vi "GraphsUpdateMain.vi"(0 "raw graph ref":refnum<vi>, 1 "File Paths":T2={"Local Save Path"=path "\\\\smbhome.uscs.susx.ac.uk\\cv222/Desktop/data", "Newton Save Path"=path "Z:/#Projects/Entanglement/data", "File Name"="test", "LocalSave"=TRUE}, 3 "Compiler Settings":T1={"Python Path"=path "", "Main File"="mainscript.py", "Meta File"="metascript.txt", "Aux File"="auxscript.py", "Pre File"="metascript.txt"}, 5 "mean graph ref":refnum<vi>, 7 "proc graph ref":refnum<vi>, 9 "ControllerSettingsRef":refnum<vi>, 11 "error in (no error)":errorcluster) -> (15 "error out":errorcluster)   [LabVIEW 2019]
uses:
  controls/FilePaths.ctl
  PulseCompiler/CompilerSettings.ctl
  controls/ControllerSettings.ctl
  controls/GlobalExp.vi
  Global.lvlib
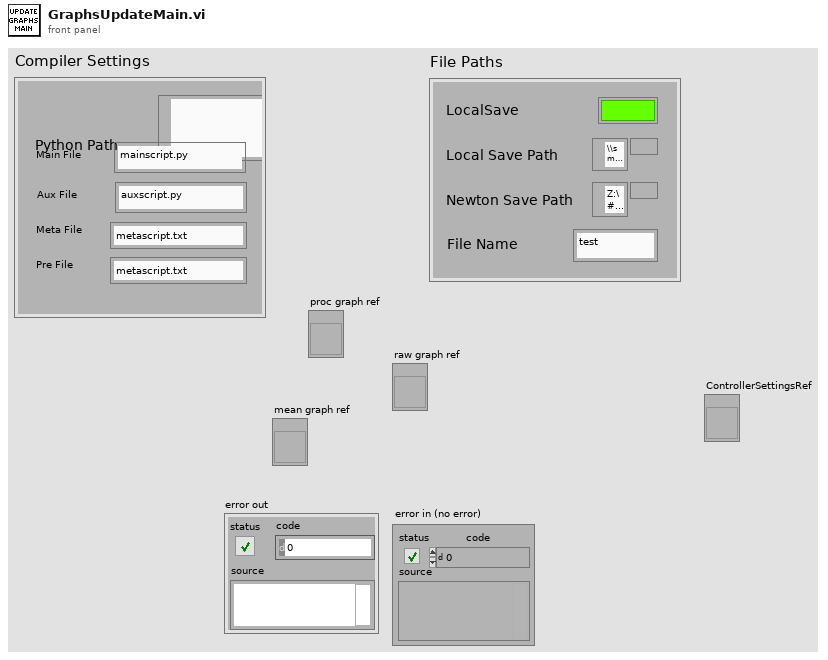
[diagram p1: front panel]
types:
  T1 = typedef "CompilerSettings.ctl" = cluster{"Python Path":path, "Main File":string, "Meta File":string, "Aux File":string, "Pre File":string}
  T2 = typedef "FilePaths.ctl" = cluster{"Local Save Path":path, "Newton Save Path":path, "File Name":string, "LocalSave":bool}
  T3 = typedef "MasterExpControl.ctl" = cluster{"Main Steps":dbl, "Main Runs":dbl, "ExpStatus":enum16{"Innit", "Stop", "Idle", "MainRunning", "AuxRunning"}, "Main Current Step":dbl, "ExpNum":dbl, "NewData":bool, "date":string, "command":string, "Stop":bool, "Pause":bool, "Mathematica":string, "Main/Meta":bool, "UpdateMath":bool, "Camera":bool, "MetaExpOver":bool, "NextMetaExp":bool}
  T4 = typedef "ControllerSettings.ctl" = cluster{"Aux Sequence":bool, "Camera":bool, "Recrystallize":bool, "Raw graph":bool, "Mean graph":bool, "Calculate probs":bool, "Find fit":bool, "ReX Time [s] :":dbl, "Lock Voltage :":dbl, "Line trig ":bool, "Check Fluo":bool, "Pre Sequence":bool}
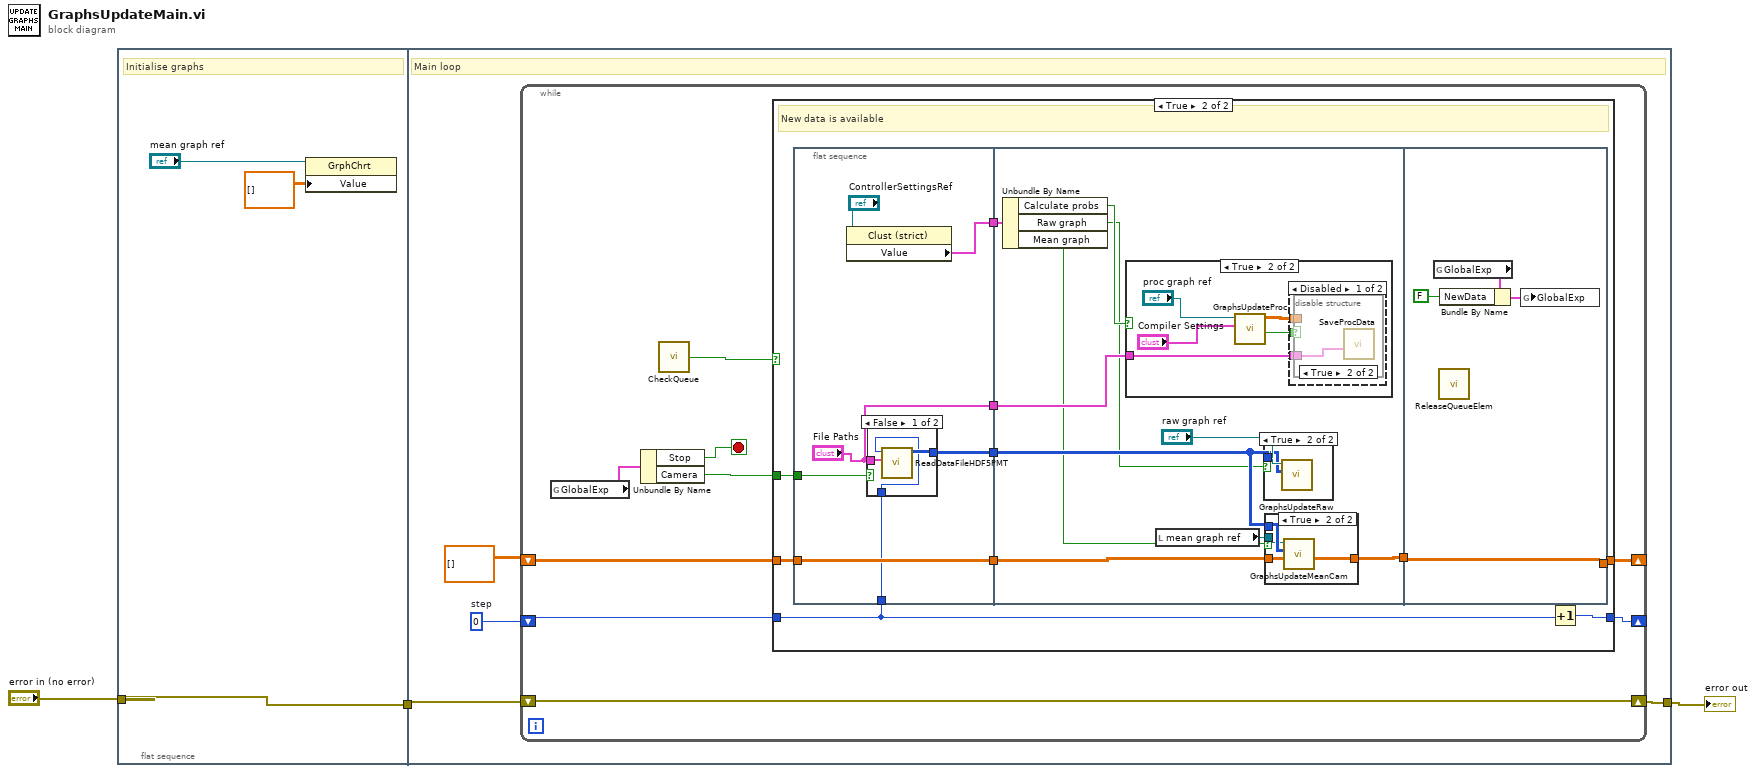
[diagram p0: block diagram]
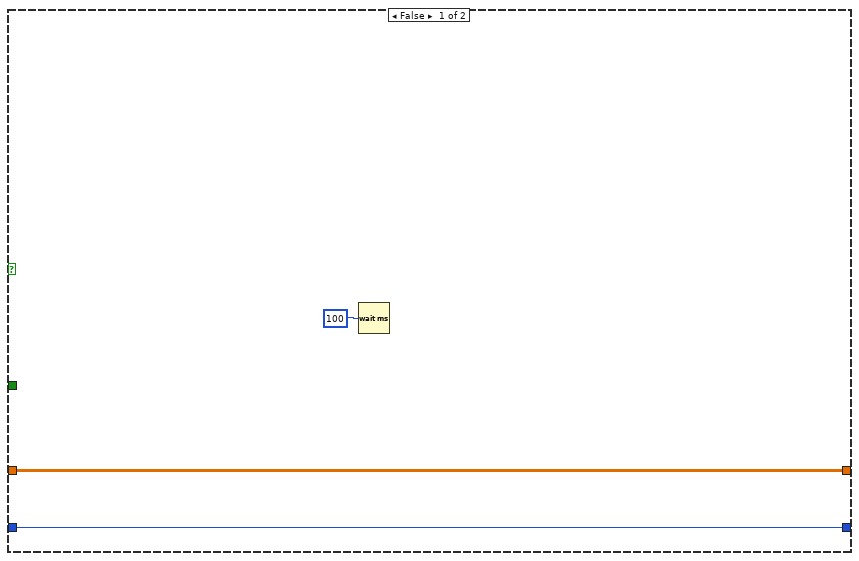
[diagram p2: hidden frame]
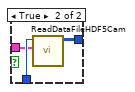
[diagram p3: hidden frame]
diagram:
  n1 = flat-sequence {
    tunnel: "error in (no error)" -> [w6]
    tunnel: [w6] -> w1
    tunnel: [w9] -> w2
    tunnel: w1 -> [w10]
    frame #0 {
      # "Initialise graphs"
      n2 = property class="GrphChrt"(reference="mean graph ref", "Value"=dbl[][] []) -> ()  [unwired: 1 in, 2 out]
    }
    frame #1 {
      w8 = 0  # step
      # "Main loop"
      n3 = while {
        shift-right: [w19] -> w9
        shift-left: w10 -> [w19]
        shift-right: [w13] -> _
        shift-left: w8 -> [w14]
        shift-right: [w11] -> _
        shift-left: dbl[][] [] -> [w12]
        stop <- w16 stop-if-true
        n4 = global read "GlobalExp.vi" "GlobalExp"() -> (w18:T3)
        n5 = Unbundle By Name(w18) -> ("Stop"=w16:bool, "Camera"=w17:bool)
        n6 = call "CheckQueue.vi"() -> ("x > 0?"=w15:bool)
        n7 = case shown="True" w15 {
          tunnel: w17 -> [_ w24]
          tunnel: w14 -> [w21 w29]
          tunnel: [w21 w32] -> w13
          tunnel: w12 -> [w20 w31]
          tunnel: [w20 w25] -> w11
          frame False {
            n8 = Wait (ms)(milliseconds to wait=u32 100) -> ()  [unwired: 1 out]
          }
          frame True {
            # "New data is available"
            n9 = flat-sequence {
              tunnel: w31 -> [w39]
              tunnel: [w39] -> w30
              tunnel: w29 -> [w38]
              tunnel: [w37] -> w28
              tunnel: ["File Paths"] -> w27
              tunnel: w24 -> [w35]
              tunnel: [w34] -> w23
              tunnel: w30 -> [w55]
              tunnel: w28 -> [w52]
              tunnel: w27 -> [w53]
              tunnel: [w50] -> w26
              tunnel: w23 -> [w48]
              tunnel: w26 -> [w72]
              tunnel: [w72] -> w25
              frame #0 {
                n10 = property class="Clust (strict)"(reference="ControllerSettingsRef") -> ("Value"=w34:T4)  [unwired: 1 in, 2 out]
                n11 = case shown="False" w35 {
                  tunnel: w38 -> [w40 w45]
                  tunnel: [w42 w44] -> w37
                  tunnel: "File Paths" -> [w41 w43]
                  frame False {
                    n12 = call "ReadDataFileHDF5PMT.vi"("File Paths"=w41, "step"=w40) -> ("last step data"=w42:i32[][])  [unwired: 8 in, 1 out]
                  }
                  frame True {
                    n13 = call "ReadDataFileHDF5Cam.vi"("File Paths"=w43, "step"=w45) -> ("last step data"=w44:i32[][])  [unwired: 8 in, 1 out]
                  }
                }
              }
              frame #1 {
                n14 = Unbundle By Name(w48) -> ("Calculate probs"=w49:bool, "Raw graph"=w47:bool, "Mean graph"=w46:bool)
                n15 = case shown="True" w49 {
                  tunnel: w53 -> [_ w57]
                  frame False {
                  }
                  frame True {
                    n16 = call "GraphsUpdateProc.vi"("Compiler Settings"="Compiler Settings", "proc graph ref"="proc graph ref") -> ("SaveToCSV?"=w59:bool, "Array"=w60:dbl[][])  [unwired: 8 in]
                    n17 = disable-structure shown="Disabled" {
                      disable-tunnel: w60 -> [w63 _]
                      disable-tunnel: w59 -> [w62 _]
                      disable-tunnel: w57 -> [w61 _]
                      frame Disabled {
                        n18 = case shown="True" w62 {
                          tunnel: w63 -> [_ _]
                          tunnel: w61 -> [_ w64]
                          frame False {
                          }
                          frame True {
                            n19 = call "SaveProcData.vi"("File Paths"=w64) -> ()  [unwired: 11 in]
                          }
                        }
                      }
                      frame Enabled {
                      }
                    }
                  }
                }
                n20 = local read "mean graph ref"() -> (w51:refnum<vi>)
                n21 = case shown="True" w47 {
                  tunnel: "raw graph ref" -> [_ w71]
                  tunnel: w52 -> [_ w70]
                  frame False {
                  }
                  frame True {
                    n22 = call "GraphsUpdateRaw.vi"("data in"=w70, "GraphChart in"=w71) -> ()  [unwired: 10 in]
                  }
                }
                n23 = case shown="True" w46 {
                  tunnel: w55 -> [w65 w69]
                  tunnel: w52 -> [_ w68]
                  tunnel: w51 -> [_ w67]
                  tunnel: [w65 w66] -> w50
                  frame False {
                  }
                  frame True {
                    n24 = call "GraphsUpdateMeanCam.vi"("Old mean data in"=w69, "run data in"=w68, "GraphChart in"=w67) -> ("New mean data out"=w66:dbl[][])  [unwired: 8 in]
                  }
                }
              }
              frame #2 {
                n25 = global read "GlobalExp.vi" "GlobalExp"() -> (w73:T3)
                n26 = call "ReleaseQueueElem.vi"() -> ()  [unwired: 12 in]
                n27 = Bundle By Name(cluster=w73, "NewData"=FALSE) -> (w74:T3)
                n28 = global write "GlobalExp.vi" "GlobalExp"(w74) -> ()
              }
            }
            n29 = Increment(x=w29) -> (x+1=w32:i32)
          }
        }
      }
    }
  }
  "error out" <- w2
